vi "Block Write.vi"(8 "error in (no error)":errorcluster, 9 "Iterations (100)":i32=100, 10 "Channel Counts":i32[](array[numeric])=[1, 10, 100, 1000, 10000, 100000], 11 "VISA resource name":refnum<visa-resource-name>) -> (0 "error out":errorcluster, 1 "Histograms":T1(array[cluster]), 2 "Metrics":T2[](array[typedef]) {"Transfer Rate" format="%.2pB/s"; "Duration Std. Dev." format="%.0f µs"; "Duration Average" format="%.0f µs"}, 3 "VISA resource name out":refnum<visa-resource-name>)   [LabVIEW 2016]
uses:
  Controls/Throughput Metrics.ctl
  <vilib>/Platform/TimedLoop/XDataNode/timing_clust.ctl
  <vilib>/Platform/TimedLoop/XDataNode/nitl_modes.ctl
  <vilib>/Platform/TimedLoop/XDataNode/wakeup.ctl
  Source/GE 5565PIORC/GE 5565PIORC.lvclass
  <vilib>/platform/TimedLoop/XDataNode/XDataNode.xnode
  <vilib>/Platform/TimedLoop/XDataNode/XDNodeRunTimeDep.lvlib
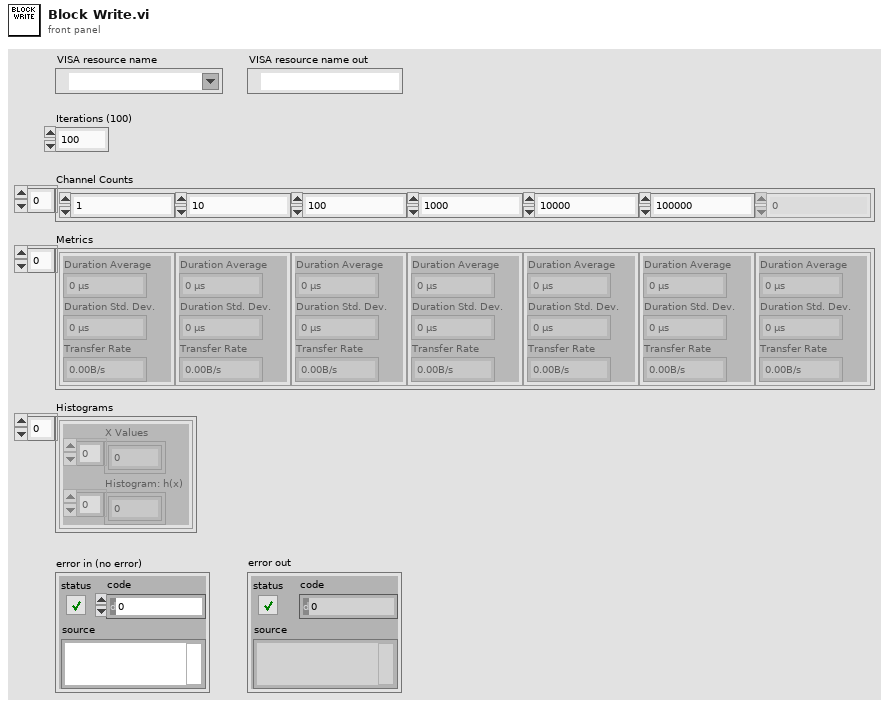
[diagram p1: front panel]
types:
  T1 = cluster{"X Values":dbl[], "Histogram: h(x)":i32[]}[]
  T2 = typedef "Throughput Metrics.ctl" = cluster{"Duration Average":u32, "Duration Std. Dev.":u32, "Transfer Rate":dbl}
  T3 = typedef "XDNodeRunTimeDep.lvlib/timing_clust.ctl" = cluster{"Expected End [f-1]":u64, "Actual End [f-1]":u64, "Finished Late? [f-1]":bool, "Expected End [i-1]":u64, "Actual End [i-1]":u64, "Finished Late? [i-1]":bool, "Expected Start [i]":u64, "Actual Start [i]":u64, "Expected Start [f]":u64, "Actual Start [f]":u64, "Source Name":string, "Structure Name":string, "Period":i64, "Deadline":i64, "Offset":i64, "Start":i64, "Priority":i32, "Timeout":i32, "Mode":T4, "Wakeup Reason":T5, "Error":errorcluster, "Source Type":string, "Secondary Source Type":string, "Global End Time":u64, "Global Start Time":u64, "Frame Duration":u64, "Iteration Duration":u64, "Assigned CPU":i32, "I/O Scan Engine Mode":u32}
  T4 = typedef "XDNodeRunTimeDep.lvlib/nitl_modes.ctl" = enum32{"No Change", "Process missed periods, maintain original phase", "Discard missed periods, maintain original phase", "Process missed periods, ignore original phase", "Discard missed periods, ignore original phase"}
  T5 = typedef "XDNodeRunTimeDep.lvlib/wakeup.ctl" = enum32{"Normal", "Aborted", "Asynchronous wakeup", "Timing source error", "Timed loop error", "Timeout"}
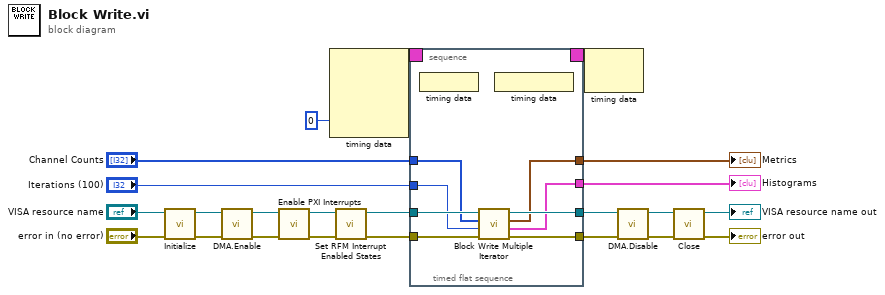
[diagram p0: block diagram]
diagram:
  n1 = call "Initialize.vi"("error in (no error)"="error in (no error)", "VISA resource name"="VISA resource name") -> ("error out"=w15:errorcluster, "GE 5565PIORC"=w16:refnum<class "GE 5565PIORC.lvclass">)  [unwired: 8 in]
  n2 = call "DMA.Enable.vi"("error in (no error)"=w15, "GE 5565PIORC in"=w16) -> ("error out"=w21:errorcluster, "GE 5565PIORC out"=w22:refnum<class "GE 5565PIORC.lvclass">)  [unwired: 8 in]
  n3 = call "Enable PXI Interrupts.vi"("error in (no error)"=w21, "GE 5565PIORC in"=w22) -> ("error out"=w19:errorcluster, "GE 5565PIORC out"=w20:refnum<class "GE 5565PIORC.lvclass">)  [unwired: 8 in]
  n4 = node-c288(0 ("Processor")) -> (w14:T3)  [unwired: 3 in]
  n5 = call "Set RFM Interrupt Enabled States.vi"("error in (no error)"=w19, "GE 5565PIORC in"=w20) -> ("error out"=w10:errorcluster, "GE 5565PIORC out"=w11:refnum<class "GE 5565PIORC.lvclass">)  [unwired: 8 in]
  n6 = timed-sequence {
    timing: w14 -> [_]
    timing-out: [_] -> w13
    tunnel: w11 -> [w31]
    tunnel: w10 -> [w30]
    tunnel: [w29] -> w9
    tunnel: [w28] -> w8
    tunnel: "Iterations (100)" -> [w27]
    tunnel: "Channel Counts" -> [w26]
    tunnel: [w25] -> w5
    tunnel: [w24] -> w2
    n7 = timed-flat-sequence {
      tunnel: w31 -> [w39]
      tunnel: w30 -> [w38]
      tunnel: [w36] -> w29
      tunnel: [w37] -> w28
      tunnel: w27 -> [w35]
      tunnel: w26 -> [w34]
      tunnel: [w33] -> w25
      tunnel: [w32] -> w24
      n8 = node-c288() -> ()  [unwired: 1 in]
      n9 = call "Block Write Multiple Iterator.vi"("error in (no error)"=w38, "Iterations (1000)"=w35, "Channel Counts"=w34, "GE 5565PIORC in"=w39) -> ("error out"=w36:errorcluster, "Histograms"=w32:T1, "Metrics"=w33:T2[], "GE 5565PIORC out"=w37:refnum<class "GE 5565PIORC.lvclass">)  [unwired: 4 in]
      n10 = node-c288() -> ()  [unwired: 1 out]
    }
  }
  "Metrics" <- w5
  "Histograms" <- w2
  n11 = node-c288(w13) -> ()  [unwired: 1 out]
  n12 = call "DMA.Disable.vi"("error in (no error)"=w9, "GE 5565PIORC in"=w8) -> ("error out"=w17:errorcluster, "GE 5565PIORC out"=w18:refnum<class "GE 5565PIORC.lvclass">)  [unwired: 8 in]
  n13 = call "Close.vi"("error in (no error)"=w17, "GE 5565PIORC in"=w18) -> ("error out"=→"error out":errorcluster, "VISA resource name out"=→"VISA resource name out":refnum<visa-resource-name>)  [unwired: 8 in]
